vi "Start Sync.vi"(8 "error in (no error)":errorcluster, 11 "OOP Server in":refnum<class "Template Server.lvclass">) -> (0 "error out":errorcluster, 3 "OOP Server out":refnum<class "Template Server.lvclass">)   [LabVIEW 2019, in "Template Server.lvlib" / "Template Server.lvclass"]
uses:
  Template Server.lvclass
  Template Server.lvclass/Template Server.ctl
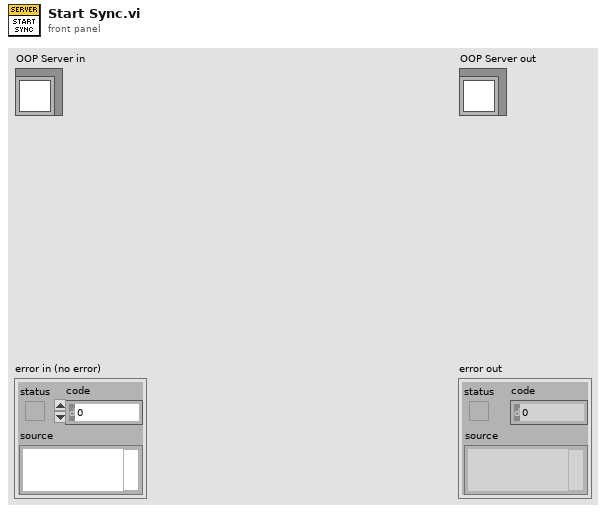
[diagram p1: front panel]
types:
  T1 = typedef "Template Server.lvlib/Template Server.lvclass/Server gRPC UEs.ctl" = cluster{"Template gRPCId UE":T2}
  T2 = typedef "gprc-lvsupport.lvlib/gRPCId Cluster UE.ctl" = refnum<user-event>
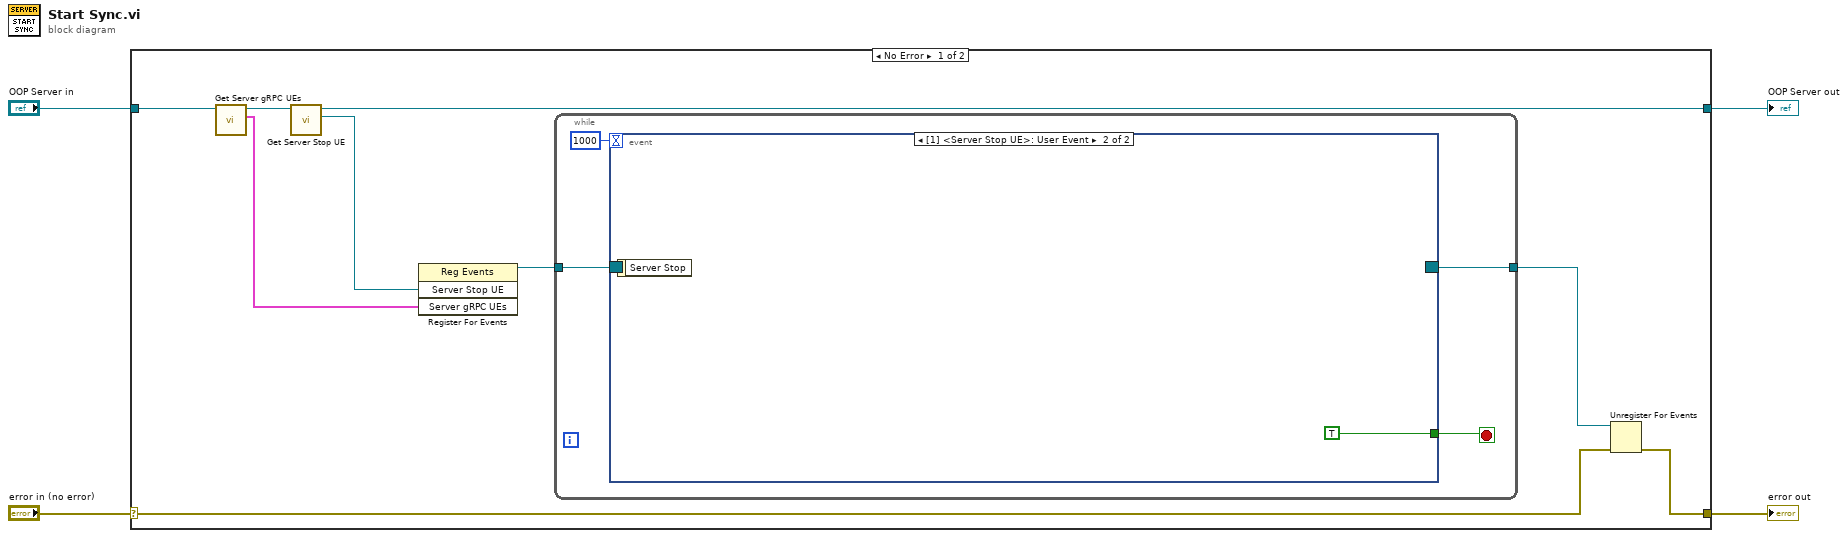
[diagram p0: block diagram]
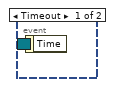
[diagram p2: hidden frame]
diagram:
  n1 = case shown="No Error" "error in (no error)" {
    selector: "error in (no error)" -> [w6 w20]
    tunnel: [w5 w20] -> w3
    tunnel: [w9 w19] -> w1
    tunnel: "OOP Server in" -> [w13 w19]
    frame No Error {
      n2 = call "Get Server gRPC UEs.vi"("OOP Server in"=w13) -> ("Server gRPC UEs"=w10:T1, "OOP Server out"=w12:refnum<class "Template Server.lvclass">)  [unwired: 9 in]
      n3 = call "Get Server Stop UE.vi"("OOP Server in"=w12) -> ("Server Stop UE"=w11:refnum<user-event>, "OOP Server out"=w9:refnum<class "Template Server.lvclass">)  [unwired: 9 in]
      n4 = register-events(w11, w10) -> (reference out=w8:refnum<event-registration>)  [unwired: 2 in, 1 out]
      n5 = while {
        tunnel: w8 -> [w17]
        tunnel: [w15] -> w7
        stop <- w16 stop-if-true
        n6 = event shown="[1] <Server Stop UE>: User Event" {
          selector: w17 -> [_ _]
          dyn-events: [_ _] -> w15
          timeout: 1000 -> [_ _]
          tunnel: [_ TRUE] -> w16
          event Timeout {
            n7 = event-data() -> ()  [unwired: 1 in, 1 out]
          }
          event User Event {
            n8 = event-data() -> ()  [unwired: 1 in, 1 out]
          }
        }
      }
      n9 = Unregister For Events(event registration refnum=w7, error in=w6) -> (error out=w5:errorcluster)
    }
    frame Error {
    }
  }
  "error out" <- w3
  "OOP Server out" <- w1
